vi "Pre-loop Init.vi"(8 "error in (no error)":errorcluster) -> (0 "error out":errorcluster, 3 "Event Registration Refnum":refnum<event-registration>)   [LabVIEW 2026, in "Error.lvlib"]
doc: "Module Initilization\nFor named purposes"
uses:
  Error.lvlib
  User Event/Event Data.ctl
  User Event/FGV Action.ctl
  Private Control/Queue FGV Action.ctl
  User Event/User Event.lvlib
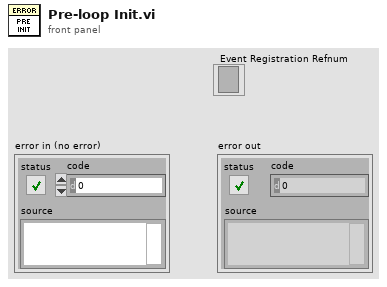
[diagram p1: front panel]
types:
  T1 = typedef "Error.lvlib/Queue FGV Action.ctl" = enum16{"Create", "Get", "Release"}
  T2 = typedef "User Event.lvlib/FGV Action.ctl" = enum16{"Create", "Get", "Destroy"}
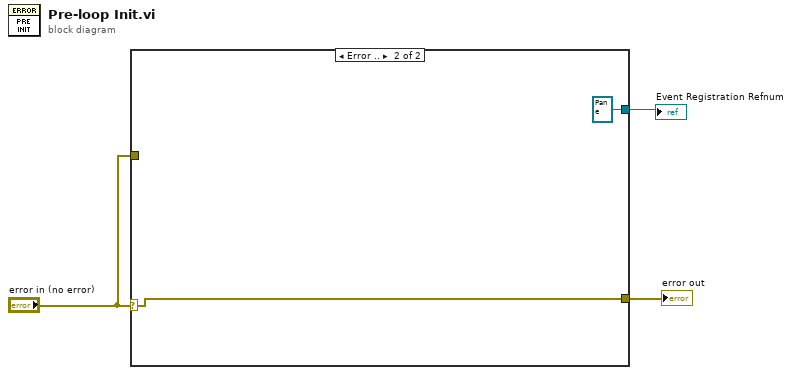
[diagram p0: block diagram]
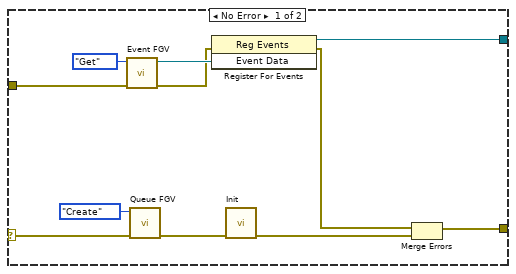
[diagram p2: hidden frame]
diagram:
  n1 = case shown="Error .." "error in (no error)" {
    selector: "error in (no error)" -> [w9 w15]
    tunnel: "error in (no error)" -> [w14 _]
    tunnel: [w5 refnum<event-registration> refnum ("Event Registration Refnum")] -> w2
    tunnel: [w4 w15] -> w1
    frame No Error {
      n2 = call "Event FGV.vi"("error in (no error)"=w14, "FGV Action"=FGV_Action."Get") -> ("error out"=w11:errorcluster, "Event Data"=w12:refnum<user-event>)  [unwired: 8 in]
      n3 = call "Queue FGV.vi"("error in (no error)"=w9, "Queue FGV  Action"=Queue_FGV_Action."Create") -> ("error out"=w8:errorcluster)  [unwired: 8 in, 1 out]
      n4 = register-events(error in=w11, w12) -> (reference out=w5:refnum<event-registration>, error out=w7:errorcluster)  [unwired: 1 in]
      n5 = call "Init.vi"("error in (no error)"=w8) -> ("error out"=w6:errorcluster)  [unwired: 10 in]
      n6 = Merge Errors(w7, w6) -> (w4:errorcluster)
    }
    frame Error {
    }
  }
  "error out" <- w1
  "Event Registration Refnum" <- w2
